vi "User Console - Fire Card Reader.vi"(8 "error in (no error)":errorcluster, 10 "Card Reader Change":bool, 11 "UE Data Container":T1) -> (0 "error out":errorcluster)   [LabVIEW 2017]
doc: "Generates Card Reader change user event."
uses:
  Shared Data/User Events/UE Data Container.ctl
  Error Handler/Controls/Error Data.ctl
  Controls/User Console - Transaction Enum.ctl
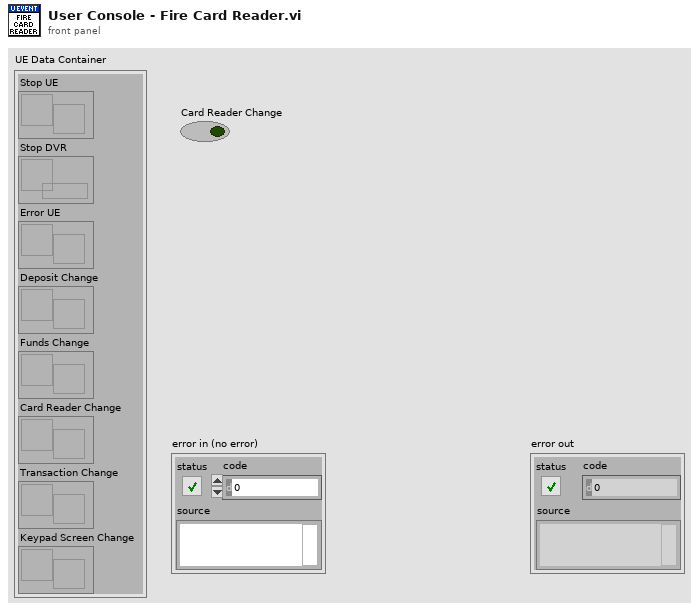
[diagram p1: front panel]
types:
  T1 = typedef "UE Data Container.ctl" = cluster{"Stop UE":refnum<user-event>, "Stop DVR":refnum<data-value>, "Error UE":refnum<user-event>, "Deposit Change":refnum<user-event>, "Funds Change":refnum<user-event>, "Card Reader Change":refnum<user-event>, "Transaction Change":refnum<user-event>, "Keypad Screen Change":refnum<user-event>}
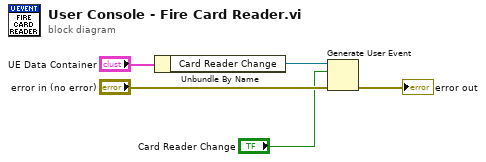
[diagram p0: block diagram]
diagram:
  n1 = Unbundle By Name("UE Data Container") -> ("Card Reader Change"=w4:refnum<user-event>)
  n2 = Generate User Event(user event=w4, event data cluster="Card Reader Change", error in="error in (no error)") -> (error out=→"error out":errorcluster)  [unwired: 1 in, 1 out]
